vi "Write Ignore Attributes.vi"(8 "error in (no error)":errorcluster, 10 "IgnoreAttributes":bool, 11 "WaveformChart.lvclass in":refnum<class "WaveformChart.lvclass">) -> (0 "error out":errorcluster, 3 "WaveformChart.lvclass out":refnum<class "WaveformChart.lvclass">)   [LabVIEW 2015, in "WaveformChart.lvclass"]
uses:
  WaveformChart.lvclass
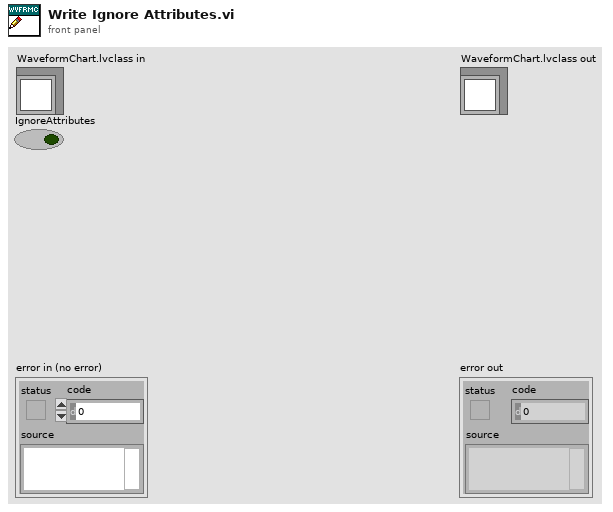
[diagram p1: front panel]
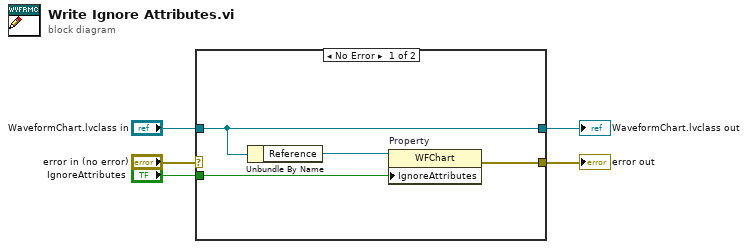
[diagram p0: block diagram]
diagram:
  n1 = case shown="No Error" "error in (no error)" {
    selector: "error in (no error)" -> [_ w11]
    tunnel: [w9 w11] -> w4
    tunnel: [w7 w10] -> w2
    tunnel: "WaveformChart.lvclass in" -> [w7 w10]
    tunnel: "IgnoreAttributes" -> [w8 _]
    frame No Error {
      n2 = Unbundle By Name(w7) -> ("Reference"=w6:refnum<vi>)
      n3 = property on="Property" class="WFChart"(reference=w6, "IgnoreAttributes"=w8) -> (error out=w9:errorcluster)  [unwired: 1 in, 1 out]
    }
    frame Error {
    }
  }
  "error out" <- w4
  "WaveformChart.lvclass out" <- w2
